vi "Straighten.vi"(8 "error in (no error)":errorcluster, 10 "Angle (rad)":dbl, 11 "Gantry in":refnum<class "A3200.lvclass">) -> (0 "error out":errorcluster, 3 "Gantry out":refnum<class "A3200.lvclass">)   [LabVIEW 2016, in "A3200.lvclass"]
uses:
  A3200.lvclass
  A3200.lvclass/A3200.ctl
  Drivers/Aerotech A3200/Motion/MoveAbsSingle.vi
  Drivers/Aerotech A3200/Aerotech VIs.lvlib
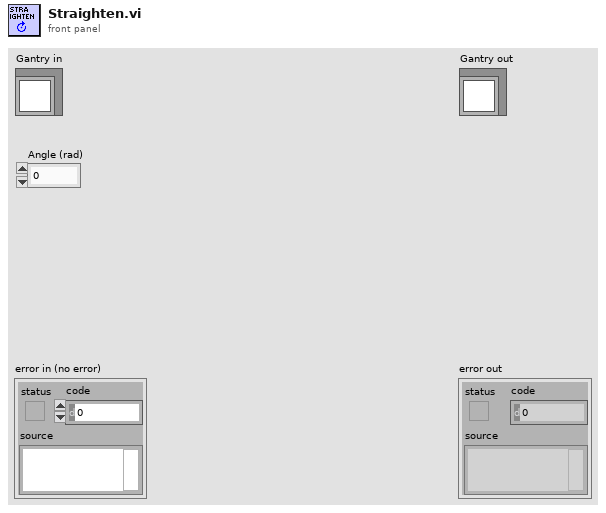
[diagram p1: front panel]
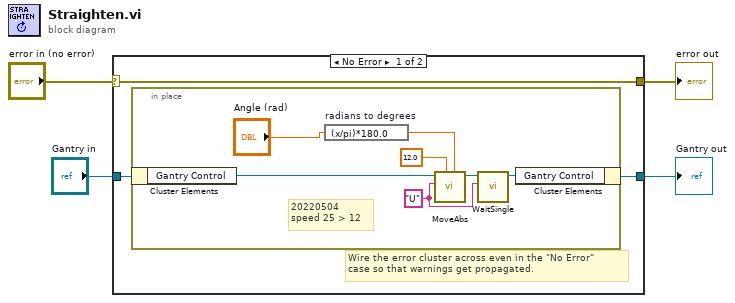
[diagram p0: block diagram]
diagram:
  n1 = case shown="No Error" "error in (no error)" {
    selector: "error in (no error)" -> [w7 w16]
    tunnel: [w7 w16] -> w3
    tunnel: [w5 w15] -> w1
    tunnel: "Gantry in" -> [w6 w15]
    frame No Error {
      # "Wire the error cluster across even in the \"No Error\"\ncase so that warnings get propagated."
      n2 = in-place {
        w12 = "U" ("element")
        # "20220504\nspeed 25 > 12"
        n3 = in-place-cluster #1(w6) -> ("Gantry Control"=w8:refnum<k24>)
        n4 = expression code="(x/pi)*180.0" "radians to degrees"("Angle (rad)") -> (w13:dbl)
        n5 = call-poly "MoveAbs.vi"("position"=w13, "speed"=12.0, "axis name"=w12, "controller in"=w8) -> ("controller out"=w11:refnum<k24>)  [unwired: 6 in, 1 out]
        n6 = call "WaitSingle.vi"("axis name"=w12, "controller in"=w11) -> ("controller out"=w9:refnum<k24>)  [unwired: 7 in, 2 out]
        n7 = in-place-cluster #1("Gantry Control"=w9) -> (w5:refnum<class "A3200.lvclass">)
      }
    }
    frame Error {
    }
  }
  "error out" <- w3
  "Gantry out" <- w1
